vi "MGI Update UI.vi"(8 "error in (no error)":errorcluster, 11 "MGI Error Handler in":refnum<class "MGI Error Reporter Dialog.lvclass">) -> (0 "error out":errorcluster, 3 "MGI Error Handler out":refnum<class "MGI Error Reporter Dialog.lvclass">)   [LabVIEW 2016, in "MGI Error Reporter Dialog.lvclass"]
doc: "This VI updates each of the 4 controls used by the MGI Error Reporter Dialog. It is called by MGI Error Reporter Dialog::Daemon at startup and when the front panel is resized.\n\nAuthored by Shawn Walpole\nsupport@mooregoodideas.com\nwww.mooregoodideas.com\n\nCopyright (c) 2013, Moore Good Ideas, Inc.\n\nAll rights reserved.\n\nRedistribution and use in source and binary forms, with or without modification, are permitted provided that the following conditions are met:\n\n * Redistributions of source code must retain the above copyright notice, this list of conditions and the following disclaimer.\n * Redistributions in binary form must reproduce the above copyright notice, this list of conditions and the following disclaimer in the documentation and/or other materials provided with the distribution.\n * Neither the name of Moore Good Ideas, Inc. nor the names of its contributors may be used to endorse or promote products derived from this software without specific prior written permission.\n\nTHIS SOFTWARE IS PROVIDED BY THE COPYRIGHT HOLDERS AND CONTRIBUTORS \"AS IS\" AND ANY EXPRESS OR IMPLIED WARRANTIES, INCLUDING, BUT NOT LIMITED TO, THE IMPLIED WARRANTIES OF MERCHANTABILITY AND FITNESS FOR A PARTICULAR PURPOSE ARE DISCLAIMED. IN NO EVENT SHALL THE COPYRIGHT OWNER OR CONTRIBUTORS BE LIABLE FOR ANY DIRECT, INDIRECT, INCIDENTAL, SPECIAL, EXEMPLARY, OR CONSEQUENTIAL DAMAGES (INCLUDING, BUT NOT LIMITED TO, PROCUREMENT OF SUBSTITUTE GOODS OR SERVICES; LOSS OF USE, DATA, OR PROFITS; OR BUSINESS INTERRUPTION) HOWEVER CAUSED AND ON ANY THEORY OF LIABILITY, WHETHER IN CONTRACT, STRICT LIABILITY, OR TORT (INCLUDING NEGLIGENCE OR OTHERWISE) ARISING IN ANY WAY OUT OF THE USE OF THIS SOFTWARE, EVEN IF ADVISED OF THE POSSIBILITY OF SUCH DAMAGE."
uses:
  <userlib>/_MGI/Error Reporter/MGI Error Reporter Dialog/MGI Error Reporter Dialog.lvclass
  <userlib>/_MGI/Application Control/MGI Set Scrollbar/MGI Set String Scrollbar.vi
  <userlib>/_MGI/Application Control/MGI Set Scrollbar/MGI Set Multicolumn Listbox Scrollbar.vi
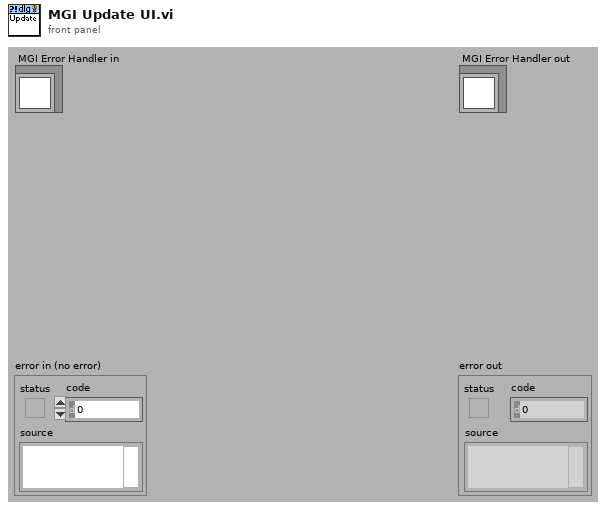
[diagram p1: front panel]
types:
  T1 = typedef "MGI Error Reporter Dialog.lvclass/MGI Dialog UI Refs Cluster.ctl" = cluster{"LB Ref":refnum<vi>, "Details Ref":refnum<vi>, "Caller Ring Ref":refnum<vi>, "Message Ref":refnum<vi>, "Clear Btn Ref":refnum<vi>}
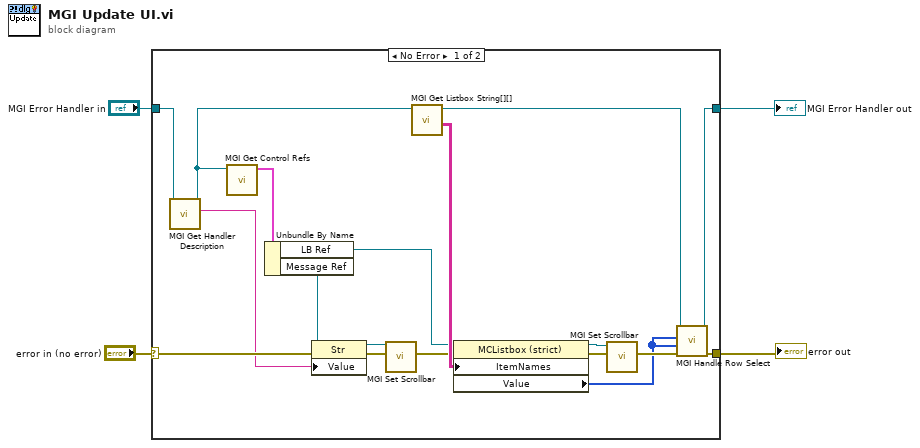
[diagram p0: block diagram]
diagram:
  n1 = case shown="No Error" "error in (no error)" {
    selector: "error in (no error)" -> [w17 w24]
    tunnel: [w8 w24] -> w3
    tunnel: [w6 w23] -> w1
    tunnel: "MGI Error Handler in" -> [w13 w23]
    frame No Error {
      n2 = call-dynamic "MGI Get Handler Description.vi"("MGI Error Handler in"=w13) -> ("Handler Description"=w16:string, "MGI Error Handler out"=w12:refnum<class "MGI Error Reporter Dialog.lvclass">)  [unwired: 1 in, 8 out]
      n3 = call <userlib>:"MGI Get Control Refs.vi"("MGI Error Dialog.lvclass"=w12) -> ("Refs"=w22:T1)  [unwired: 10 out]
      n4 = Unbundle By Name(w22) -> ("LB Ref"=w10:refnum<vi>, "Message Ref"=w18:refnum<vi>)
      n5 = property class="Str"(reference=w18, error in=w17, "Value"=w16) -> (reference out=w15:refnum<vi>, error out=w14:errorcluster)
      n6 = call-poly <userlib>:"MGI Set Scrollbar.vi"("Error In"=w14, "String Reference"=w15) -> ("Error Out"=w11:errorcluster)  [unwired: 9 out]
      n7 = call-dynamic "MGI Get Listbox String[][].vi"("MGI Error Dialog in"=w12) -> ("Error[Row][Err/Warn,Name,Time,Count]"=w19:string[][], "MGI Error Dialog out"=w7:refnum<class "MGI Error Reporter Dialog.lvclass">)  [unwired: 2 in, 7 out]
      n8 = property class="MCListbox (strict)"(reference=w10, error in=w11, "ItemNames"=w19) -> (reference out=w21:refnum<vi>, error out=w20:errorcluster, "Value"=w5:i32[])
      n9 = call-poly <userlib>:"MGI Set Scrollbar.vi"("Error In"=w20, "Listbox Reference In"=w21) -> ("Error Out"=w9:errorcluster)  [unwired: 9 out]
      n10 = call-dynamic "MGI Handle Row Select.vi"("error in (no error)"=w9, "Old Selected[]"=w5, "Selected[]"=w5, "MGI Error Handler in"=w7) -> ("error out"=w8:errorcluster, "MGI Error Handler out"=w6:refnum<class "MGI Error Reporter Dialog.lvclass">)  [unwired: 6 out]
    }
    frame Error {
    }
  }
  "error out" <- w3
  "MGI Error Handler out" <- w1
